vi "Vol-Viewer UI initialisation.vi"(5 "Source number of frames":T2(ring), 8 "error in (no error)":errorcluster) -> (0 "error out":errorcluster, 1 "VL array refs":T1[](array[typedef]), 2 "Number of Frames":u32, 3 "Image ref":T1, 4 "Scrollbar position":i32)   [LabVIEW 2020]
uses:
  <vilib>/vision/Image Controls.llb/IMAQ Image.ctl
  Timelapse Viewer/Globals/gl_Time series viewer globals.vi
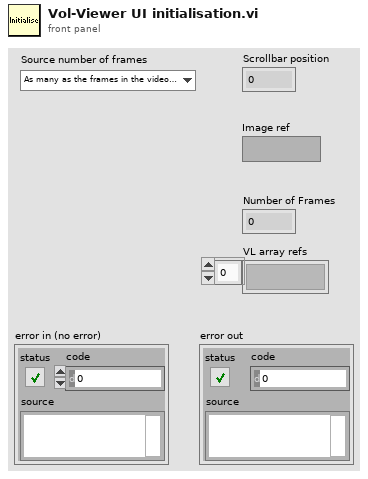
[diagram p1: front panel]
types:
  T1 = typedef "IMAQ Image.ctl" = refnum<image>
  T2 = enum16{"As many as the frames in the video with the fewest frames", "As many as the number of cycles"}
  T3 = enum8{"Enabled", "Disabled", "Disabled and Grayed Out"}
  T4 = typedef "Time series viewer refs.ctl" = cluster{"This VI":refnum<vi>, "Image control":refnum<vi>, "AVI Mode ind":refnum<vi>, "Play":refnum<vi>, "Stop":refnum<vi>, "Back":refnum<vi>, "Scrollbar":refnum<vi>, "Video length info":refnum<vi>, "Expected speed values":refnum<vi>, "Intensity":refnum<vi>, "Path":refnum<vi>, "Selection sliders":refnum<vi>, "Speed Graph ref":refnum<vi>, "Frame rate set (fps)":refnum<vi>, "Number of rows to generate":refnum<vi>, "VL Image Array":refnum<vi>, "Image Scrollbar":refnum<vi>, "Channel to load":refnum<vi>, "Colour":refnum<vi>}
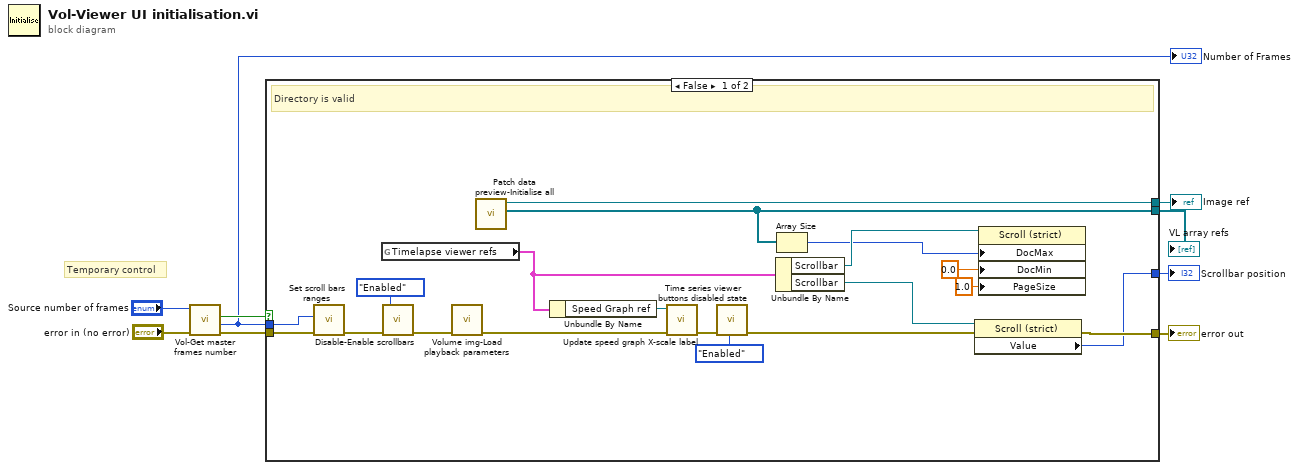
[diagram p0: block diagram]
diagram:
  # "Temporary control"
  n1 = call "Vol-Get master frames number.vi"("Source number of frames"="Source number of frames", "error in (no error)"="error in (no error)") -> ("error out"=w8:errorcluster, "Number of Frames"=w5:u32, "Cancelled due to the selected \nAVI file being located within an\n\"Exported 8-bit videos\" directory!"=w6:bool)  [unwired: 6 in, 1 out]
  "Number of Frames" <- w5
  n2 = case shown="False" w6 {
    tunnel: w8 -> [w29 w30]
    tunnel: w5 -> [w28 _]
    tunnel: [w27 w30] -> w7
    tunnel: [w26 _] -> w3
    tunnel: [w25 _] -> w2
    tunnel: [w12 _] -> w1
    frame False {
      # "Directory is valid"
      n3 = call "Set scroll bars ranges.vi"("error in (no error)"=w29, "Number of frames"=w28) -> ("error out"=w15:errorcluster)  [unwired: 9 in]
      n4 = global read "gl_Time series viewer globals.vi" "Timelapse viewer refs"() -> (w20:T4)
      n5 = call "Disable-Enable scrollbars.vi"("error in (no error)"=w15, "Disabled state"=T3."Enabled") -> ("error out"=w23:errorcluster)  [unwired: 9 in]
      n6 = call "Volume img-Load playback parameters.vi"("error in (no error)"=w23) -> ("error out"=w19:errorcluster)  [unwired: 9 in, 1 out]
      n7 = call "Patch data preview-Initialise all.vi"() -> ("VL array refs"=w12:T1[], "U8 Image ref"=w25:T1)  [unwired: 10 in]
      n8 = Unbundle By Name(w20) -> ("Speed Graph ref"=w22:refnum<vi>)
      n9 = call "Update speed graph X-scale label.vi"("error in (no error)"=w19, "Speed Graph"=w22) -> ("error out"=w17:errorcluster)  [unwired: 9 in]
      n10 = call "Time series viewer buttons disabled state.vi"("error in (no error)"=w17, "Disabled"=T3."Enabled") -> ("error out"=w16:errorcluster)  [unwired: 9 in]
      n11 = Unbundle By Name(w20) -> ("Scrollbar"=w14:refnum<vi>, "Scrollbar"=w21:refnum<vi>)
      n12 = Array Size(array=w12) -> (size(s)=w11:i32)
      n13 = property class="Scroll (strict)"(reference=w21, error in=w16) -> (error out=w27:errorcluster, "Value"=w26:i32)  [unwired: 1 out]
      n14 = property class="Scroll (strict)"(reference=w14, "DocMax"=w11, "DocMin"=0.0 ("Doc Min"), "PageSize"=1.0 ("Page Size")) -> ()  [unwired: 1 in, 2 out]
    }
    frame True {
      # "Cancelled due to the selected AVI file being located within an \"Exported 8-bit videos\" directory!"
    }
  }
  "error out" <- w7
  "Scrollbar position" <- w3
  "Image ref" <- w2
  "VL array refs" <- w1
